vi "DataFinder Name.vi"(3 "Default Name (My DataFinder)":string="My DataFinder") -> (1 "DataFinder Name":string)   [LabVIEW 2011]
uses:
  server lib/Spartan CONFIG Global.vi
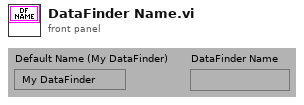
[diagram p1: front panel]
types:
  T1 = typedef "Keyed Array.ctl" = cluster{"keys":string[], "values":string[]}
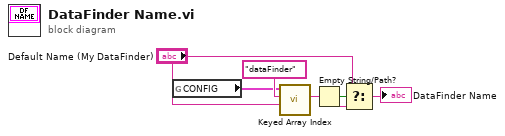
[diagram p0: block diagram]
diagram:
  n1 = global read "Spartan CONFIG Global.vi" "CONFIG"() -> (w5:T1)
  n2 = call "Keyed Array Index.vi"("default value"="Default Name (My DataFinder)", "key"="dataFinder", "array in"=w5) -> ("value"=w3:string)  [unwired: 1 in, 3 out]
  n3 = Empty String/Path?(string/path=w3) -> (empty?=w4:bool)
  n4 = Select(t="Default Name (My DataFinder)", s=w4, f=w3) -> (s? t:f=→"DataFinder Name":string)
